vi "_DRIVER_SHARED_Get Driver Controls on Connector Pane.vi"(8 "error in (no error)":errorcluster, 11 "Path of [...]_driver.vi":path=path "C:/UG-WORK/_DRIVER_/LV2020/NI9205/NI9205_driver.vi") -> (0 "error out":errorcluster, 1 "String Control Variables":T1[](array[typedef]), 2 "Ctrls Array":variant[](array[variant]), 3 "Ctrls ref":refnum<vi>[](array[refnum]), 5 "VI Reference":refnum<vi>)   [LabVIEW 2020]
doc: "GET CONTROLS ON CONNECTOR PANE AND CONVERT VALUES INTO STRING"
uses:
  TYPEDEF/_DRIVER_SHARED_TYPEDEF_StringControlVaviables.ctl
panel:
  out "Control Names":string[](array[string])
  out "Type":string[](array[string])
  out "Indicator Names":string[](array[string])
  # "GET CONTROLS ON CONNECTOR PANE AND CONVERT VALUES INTO STRING"
  # "INPUT"
  # "OUTPUT"
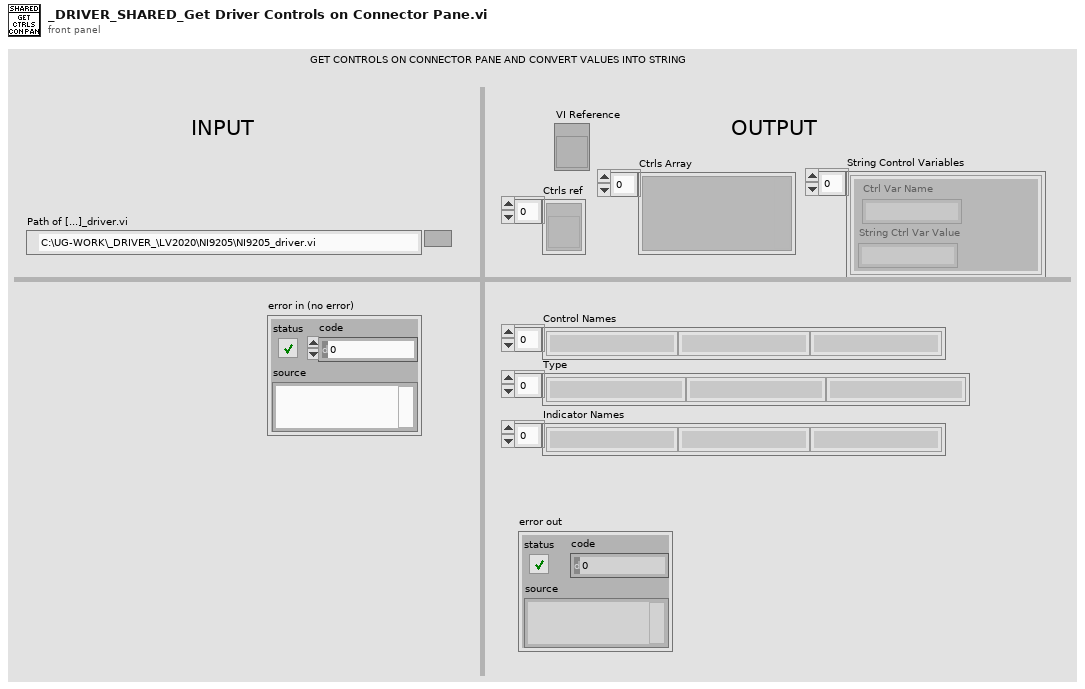
[diagram p1: front panel]
types:
  T1 = typedef "_DRIVER_SHARED_TYPEDEF_StringControlVaviables.ctl" = cluster{"Ctrl Var Name":string, "String Ctrl Var Value":string}
  T2 = cluster{"Show Names":bool, "Hide Root Name":bool, "Enums as String":bool, "ISO8601 Timestamps":bool}
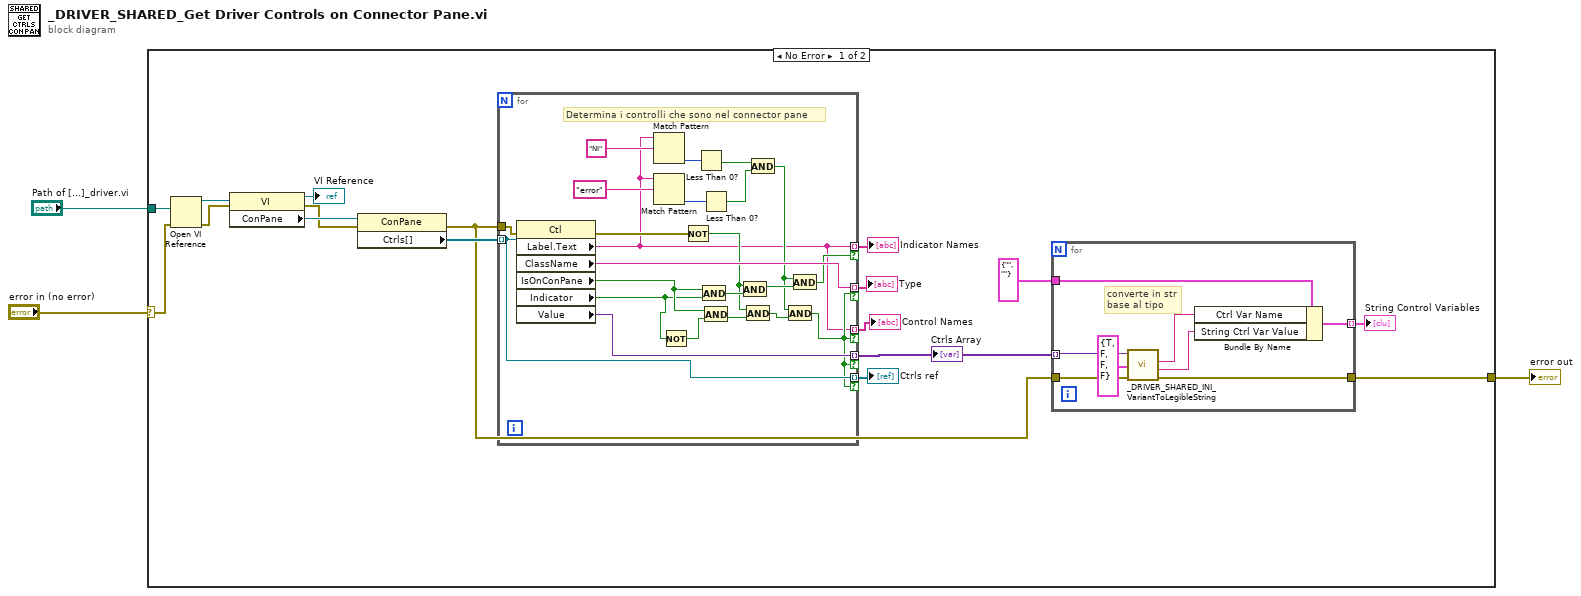
[diagram p0: block diagram]
diagram:
  n1 = case shown="No Error" "error in (no error)" {
    selector: "error in (no error)" -> [w8 w52]
    tunnel: "Path of [...]_driver.vi" -> [w18 _]
    tunnel: [w7 w52] -> w1
    frame No Error {
      n2 = Open VI Reference(vi path=w18, error in (no error)=w8) -> (vi reference=w19:refnum<vi>, error out=w17:errorcluster)  [unwired: 4 in]
      n3 = property class="VI"(reference=w19, error in=w17) -> (reference out=→"VI Reference":refnum<vi>, error out=w16:errorcluster, "ConPane"=w20:refnum<vi>)
      n4 = property class="ConPane"(reference=w20, error in=w16) -> (error out=w9:errorcluster, "Ctrls[]"=w11:refnum<vi>[])  [unwired: 1 out]
      n5 = for {
        tunnel: [w31] -> w15 mode=indexing if=w32
        tunnel: w11 -> [w43] mode=indexing
        tunnel: [w51] -> w14 mode=indexing if=w40
        tunnel: [w31] -> w12 mode=indexing if=w40
        tunnel: [w44] -> w10 mode=indexing if=w40
        tunnel: [w43] -> w13 mode=indexing if=w40
        tunnel: w9 -> [w35]
        # "Determina i controlli che sono nel connector pane"
        n6 = property class="Ctl"(reference=w43, error in=w35) -> (error out=w46:errorcluster, "Label.Text"=w31:string, "ClassName"=w51:string, "IsOnConPane"=w49:bool, "Indicator"=w47:bool, "Value"=w44:variant)  [unwired: 1 out]
        n7 = Match Pattern(string=w31, regular expression="NI") -> (offset past match=w38:i32)  [unwired: 1 in, 3 out]
        n8 = Match Pattern(string=w31, regular expression="error") -> (offset past match=w41:i32)  [unwired: 1 in, 3 out]
        n9 = Not(x=w47) -> (.not. x?=w48:bool)
        n10 = Not(x=w46) -> (.not. x?=w45:bool)
        n11 = Less Than 0?(x=w38) -> (x < 0?=w36:bool)
        n12 = And(x=w49, y=w47) -> (x .and. y?=w50:bool)
        n13 = Less Than 0?(x=w41) -> (x < 0?=w37:bool)
        n14 = And(x=w49, y=w48) -> (x .and. y?=w29:bool)
        n15 = And(x=w45, y=w50) -> (x .and. y?=w34:bool)
        n16 = And(x=w45, y=w29) -> (x .and. y?=w30:bool)
        n17 = And(x=w36, y=w37) -> (x .and. y?=w33:bool)
        n18 = And(x=w33, y=w30) -> (x .and. y?=w40:bool)
        n19 = And(x=w33, y=w34) -> (x .and. y?=w32:bool)
      }
      "Indicator Names" <- w15
      "Type" <- w14
      "Control Names" <- w12
      "Ctrls Array" <- w10
      "Ctrls ref" <- w13
      n20 = for {
        tunnel: w10 -> [w28] mode=indexing
        tunnel: w9 -> [w27]
        tunnel: [w26] -> w7
        tunnel: T1 {"Ctrl Var Name"="", "String Ctrl Var Value"=""} ("String Control Variables") -> [w24]
        tunnel: [w21] -> w5 mode=indexing
        # "converte in str\nbase al tipo"
        n21 = call "_DRIVER_SHARED_INI_VariantToLegibleString.vi"("Format Options"=T2 {"Show Names"=TRUE, "Hide Root Name"=FALSE, "Enums as String"=FALSE, "ISO8601 Timestamps"=FALSE}, "error in (no error)"=w27, "Variant"=w28) -> ("error out"=w26:errorcluster, "Var_Value"=w22:string, "Var_name"=w23:string)  [unwired: 5 in, 1 out]
        n22 = Bundle By Name(cluster=w24, "Ctrl Var Name"=w23, "String Ctrl Var Value"=w22) -> (w21:T1)
      }
      "String Control Variables" <- w5
    }
    frame Error {
    }
  }
  "error out" <- w1
